vi "Transient Memory (Store).vi"(6 "Settle (1mS)":u32=1, 8 "error in (no error)":errorcluster, 9 "Save Memory ( 1)":i32=1, 10 "Save Mode (0: List)":u16(ring) items=["List", "Wave"], 11 "VISA resource name":refnum<visa-resource-name>) -> (0 "error out":errorcluster, 3 "VISA resource name out":refnum<visa-resource-name>)   [LabVIEW 2018, in "TDK-Lambda Z.lvlib"]
doc: "Saves <1..4> the last selected List/Wave type (voltage or/and current) , type values and time values from volatile memory\n\nNote: List and Wave store in cell are same. So when data stored in cell <n> in Wave it overwrite on data stored in List with same number"
uses:
  TDK-Lambda Z.lvlib
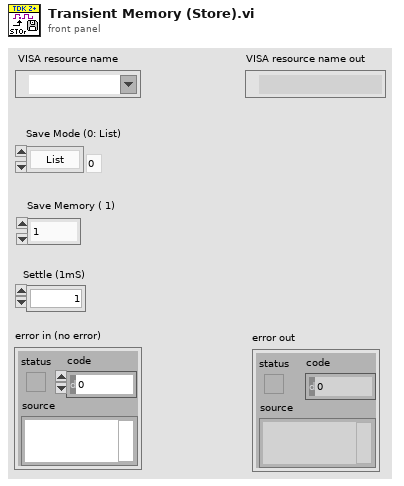
[diagram p1: front panel]
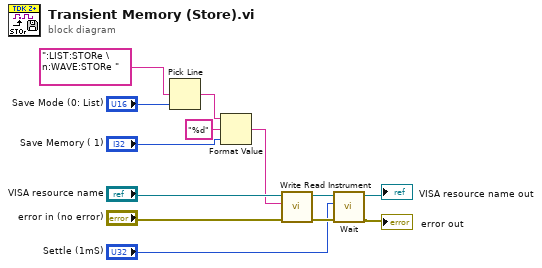
[diagram p0: block diagram]
diagram:
  n1 = Pick Line(multi-line string=":LIST:STORe \n:WAVE:STORe ", line index="Save Mode (0: List)") -> (output string=w2:string)  [unwired: 1 in]
  n2 = Format Value(string ("")=w2, format string="%d", value (0)="Save Memory ( 1)") -> (output string=w5:string)
  n3 = call "Write Read Instrument.vi"("error in (no error)"="error in (no error)", "SCPI  Write Command/Query"=w5, "VISA resource name"="VISA resource name") -> ("error out"=w10:errorcluster, "VISA resource name out"=w11:refnum<visa-resource-name>)  [unwired: 6 in, 1 out]
  n4 = call "Wait.vi"("error in (no error)"=w10, "Wait (1mS)"="Settle (1mS)", "VISA resource name"=w11) -> ("error out"=→"error out":errorcluster, "VISA resource name out"=→"VISA resource name out":refnum<visa-resource-name>)  [unwired: 7 in]
